vi "GetProxy.vi"(8 "error in (no error)":errorcluster, 11 "Enum":enum16{"Subject 1", "Subject 2"}(ring)) -> (0 "error out":errorcluster, 3 "OperationLogger (proxy) out":refnum<class "OperationLogger (proxy).lvclass">)   [LabVIEW 2014, in "Normal Proxy.lvlib" / "OperationLogger (proxy).lvclass"]
uses:
  OperationLogger (proxy).lvclass
  OperationLogger (proxy).lvclass/OperationLogger (proxy).ctl
  Normal Proxy.lvlib
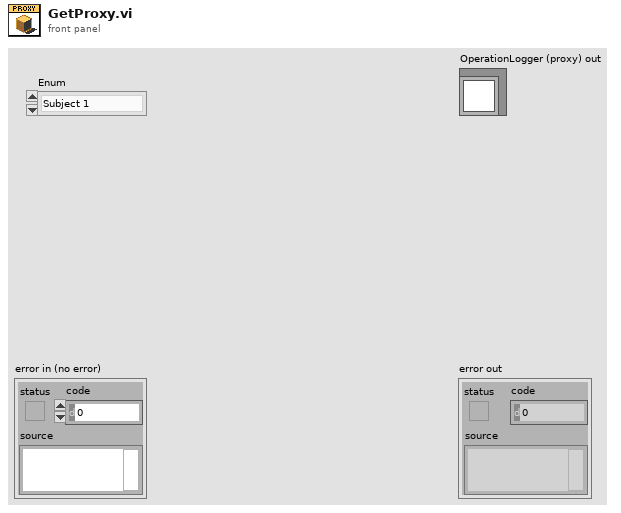
[diagram p1: front panel]
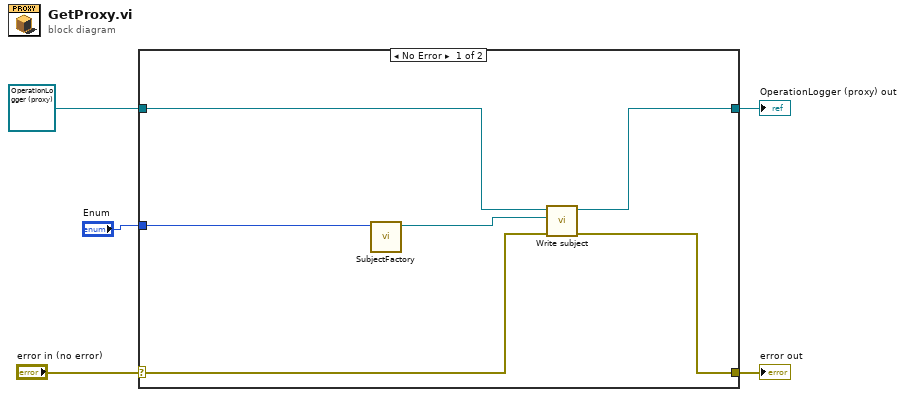
[diagram p0: block diagram]
diagram:
  n1 = case shown="No Error" "error in (no error)" {
    selector: "error in (no error)" -> [w7 w13]
    tunnel: [w6 w13] -> w4
    tunnel: [w8 w12] -> w2
    tunnel: refnum<class "OperationLogger (proxy).lvclass"> refnum ("OperationLogger (proxy) in") -> [w9 w12]
    tunnel: "Enum" -> [w11 _]
    frame No Error {
      n2 = call "SubjectFactory.vi"("Enum"=w11) -> ("Normal Proxy.lvlib:Subject.lvclass"=w10:refnum<class "Subject.lvclass">)  [unwired: 10 in]
      n3 = call "Write subject.vi"("error in (no error)"=w7, "Normal Proxy.lvlib:Subject.lvclass"=w10, "OperationLogger (proxy) in"=w9) -> ("error out"=w6:errorcluster, "OperationLogger (proxy) out"=w8:refnum<class "OperationLogger (proxy).lvclass">)  [unwired: 7 in]
    }
    frame Error {
    }
  }
  "error out" <- w4
  "OperationLogger (proxy) out" <- w2
